vi "job3.vi"(8 "error in (no error)":errorcluster, 11 "Worker3(receiver) in":refnum<class "Worker3(receiver).lvclass">) -> (0 "error out":errorcluster, 3 "Worker3(receiver) out":refnum<class "Worker3(receiver).lvclass">)   [LabVIEW 2014, in "Worker3(receiver).lvclass"]
uses:
  Worker3(receiver).lvclass
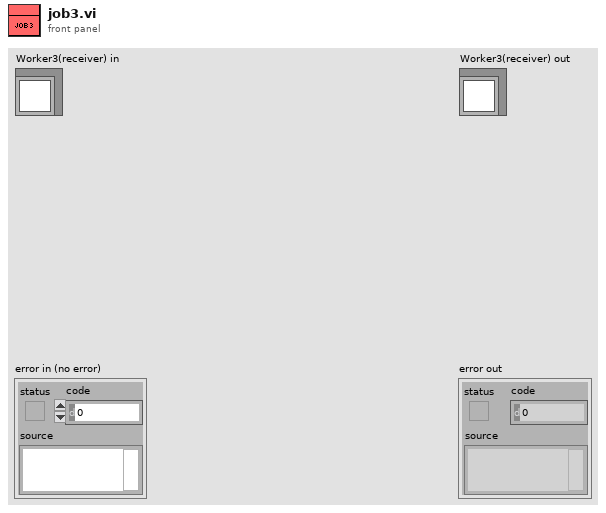
[diagram p1: front panel]
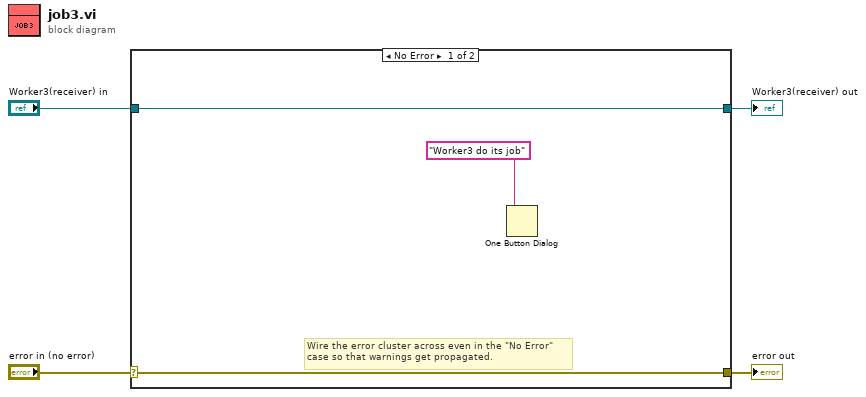
[diagram p0: block diagram]
diagram:
  n1 = case shown="No Error" "error in (no error)" {
    selector: "error in (no error)" -> [w6 w9]
    tunnel: [w6 w9] -> w3
    tunnel: [w7 w8] -> w1
    tunnel: "Worker3(receiver) in" -> [w7 w8]
    frame No Error {
      # "Wire the error cluster across even in the \"No Error\"\ncase so that warnings get propagated."
      n2 = One Button Dialog(message="Worker3 do its job") -> ()  [unwired: 1 in, 1 out]
    }
    frame Error {
    }
  }
  "error out" <- w3
  "Worker3(receiver) out" <- w1
